vi "Initialize.vi"(8 "error in (no error)":errorcluster, 9 "Requestor":string, 10 "Requestee":string, 11 "Mag Lab Hardware in":refnum<class "Mag Lab Measure Base.lvclass">) -> (0 "error out":errorcluster, 3 "Mag Lab Hardware out":refnum<class "Mag Lab Measure Base.lvclass">)   [LabVIEW 2015, in "Mag Lab Measure Base.lvclass"]
uses:
  Mag Lab Measure Base.lvclass
  Mag Lab Root/Mag Lab Root.lvclass/Mag Lab Root.ctl
  Mag Lab Properties/Mag Lab Parameters.lvclass
  Mag Lab Root/Mag Lab Root.lvclass
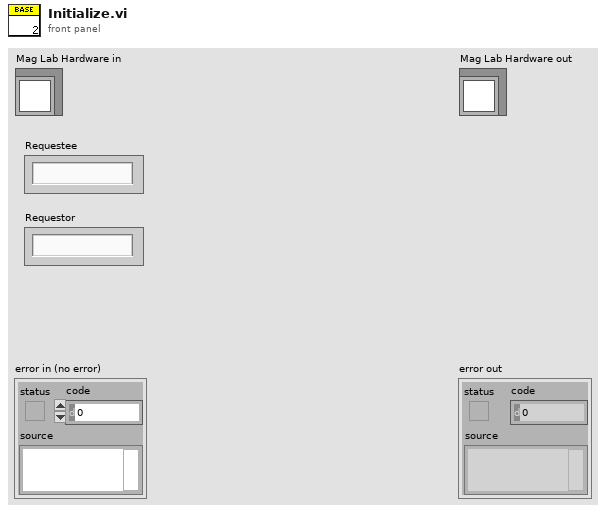
[diagram p1: front panel]
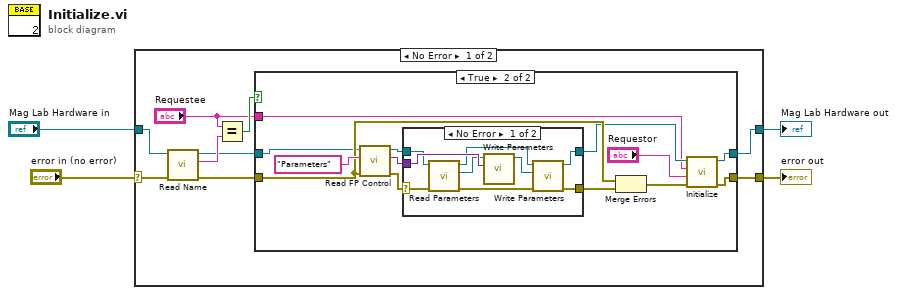
[diagram p0: block diagram]
diagram:
  n1 = case shown="No Error" "error in (no error)" {
    selector: "error in (no error)" -> [w10 w40]
    tunnel: [w13 w40] -> w3
    tunnel: [w12 w39] -> w1
    tunnel: "Mag Lab Hardware in" -> [w11 w39]
    frame No Error {
      n2 = call "Read Name.vi"("error in (no error)"=w10, "Mag Lab Root in"=w11) -> ("error out"=w8:errorcluster, "Name"=w9:string, "Mag Lab Root out"=w5:refnum<class "Mag Lab Measure Base.lvclass">)  [unwired: 7 in]
      n3 = Equal?(x="Requestee", y=w9) -> (x = y?=w7:bool)
      n4 = case shown="True" w7 {
        tunnel: [w15 w21] -> w13
        tunnel: [w14 w19] -> w12
        tunnel: w8 -> [w15 w22]
        tunnel: "Requestee" -> [_ w18]
        tunnel: w5 -> [w14 w16]
        frame False {
        }
        frame True {
          n5 = call-dynamic "Read FP Control.vi"("error in (no error)"=w22, "Control Name"="Parameters", "Mag Lab Measure Base in"=w16) -> ("error out"=w27:errorcluster, "Control Value"=w26:variant, "Mag Lab Measure Base out"=w25:refnum<class "Mag Lab Measure Base.lvclass">)  [unwired: 6 in]
          n6 = case shown="No Error" w27 {
            selector: w27 -> [w30 _]
            tunnel: w26 -> [w35 _]
            tunnel: w25 -> [w33 w38]
            tunnel: [w37 _] -> w24
            tunnel: [w36 w38] -> w20
            frame No Error {
              n7 = call-dynamic "Read Parameters.vi"("error in (no error)"=w30, "Mag Lab Root in"=w33) -> ("error out"=w29:errorcluster, "Mag Lab Parameters.lvclass"=w31:refnum<class "Mag Lab Parameters.lvclass">, "Mag Lab Root out"=w32:refnum<class "Mag Lab Measure Base.lvclass">)  [unwired: 7 in]
              n8 = call-dynamic "Write Parameters.vi"("Parameters"=w35, "Mag Lab Parameters in"=w31) -> ("Mag Lab Parameters out"=w34:refnum<class "Mag Lab Parameters.lvclass">)  [unwired: 8 in, 1 out]
              n9 = call-dynamic "Write Parameters.vi"("error in (no error)"=w29, "Mag Lab Parameters.lvclass"=w34, "Mag Lab Root in"=w32) -> ("error out"=w37:errorcluster, "Mag Lab Root out"=w36:refnum<class "Mag Lab Measure Base.lvclass">)  [unwired: 7 in]
            }
            frame Error {
            }
          }
          n10 = Merge Errors(w22, w24) -> (w23:errorcluster)
          n11 = call-parent "Initialize.vi"("error in (no error)"=w23, "Requestor"="Requestor", "Requestee"=w18, "Mag Lab Root in"=w20) -> ("error out"=w21:errorcluster, "Mag Lab Root out"=w19:refnum<class "Mag Lab Measure Base.lvclass">)  [unwired: 6 in]
        }
      }
    }
    frame Error {
    }
  }
  "error out" <- w3
  "Mag Lab Hardware out" <- w1
